vi "I64 to U32 and Error.vi"(4 "error in (no error)":errorcluster, 6 "U64":dbl) -> (0 "error out":errorcluster, 2 "U32":u32 format="%.0x", 3 "Error if <0":i32 format="%.0x")   [LabVIEW 2017]
panel:
  # "LVHDF5 Toolkit\nCopyright (c) 2005-2013 by Jason D. Sommerville\nCopyright (c) 2014 by UPVI, LLC.\n\nThis use and distribution of this file is governed by the terms found in \nLICENSE.txt distributed with this toolkit and installed at\n <user.lib>\\_lvhdf5\\LICENSE.txt"
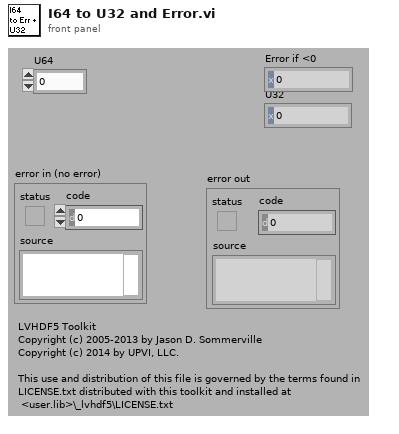
[diagram p1: front panel]
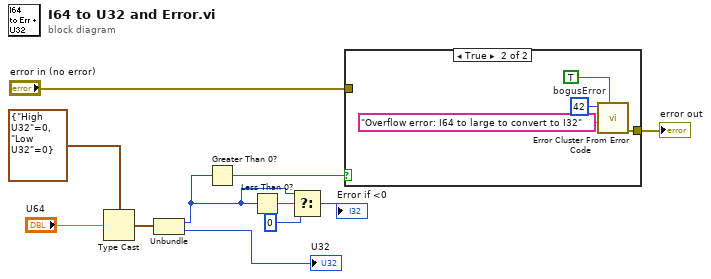
[diagram p0: block diagram]
diagram:
  n1 = Type Cast(type=cluster{"High U32":i32, "Low U32":u32} {"High U32"=0, "Low U32"=0}, x="U64") -> (*(type *) &x=w9:cluster{"High U32":i32, "Low U32":u32})
  n2 = Unbundle(w9) -> ("High U32"=w3:i32, "Low U32"=→"U32":u32)
  n3 = Greater Than 0?(x=w3) -> (x > 0?=w5:bool)
  n4 = Less Than 0?(x=w3) -> (x < 0?=w4:bool)
  n5 = Select(t=w3, s=w4, f=0) -> (s? t:f=→"Error if <0":i32)
  n6 = case shown="True" w5 {
    tunnel: [w12 w13] -> w8
    tunnel: "error in (no error)" -> [w12 _]
    frame False {
    }
    frame True {
      w16 = 42  # bogusError
      n7 = call <vilib>:"Error Cluster From Error Code.vi"("show call chain? (False)"=TRUE, "error message (\"\")"="Overflow error: I64 to large to convert to I32" ("error message (\"\")"), "error code (0)"=w16) -> ("error out"=w13:errorcluster)  [unwired: 6 in]
    }
  }
  "error out" <- w8
